vi "Shutdown.vi"(8 "error in (no error)":errorcluster, 11 "GRMActor in":refnum<class "GRMActor.lvclass">) -> (0 "error out":errorcluster, 3 "GRMActor out":refnum<class "GRMActor.lvclass">)   [LabVIEW 2020, in "GRMActor.lvlib" / "GRMActor.lvclass"]
uses:
  GRMActor.lvclass
  GRMActor.lvclass/GRMActor.ctl
  <vilib>/ActorFramework/Message Enqueuer/Message Enqueuer.lvclass/Message Enqueuer.ctl
  <vilib>/ActorFramework/Message Enqueuer/Enqueue.vi
  <vilib>/ActorFramework/Stop Msg/Stop Msg.lvclass
  C:/Program Files/National Instruments/LabVIEW 2020/vi.lib/ActorFramework/Message/Message.lvclass
  <vilib>/ActorFramework/Message Priority Queue/Priority Enqueue.vi
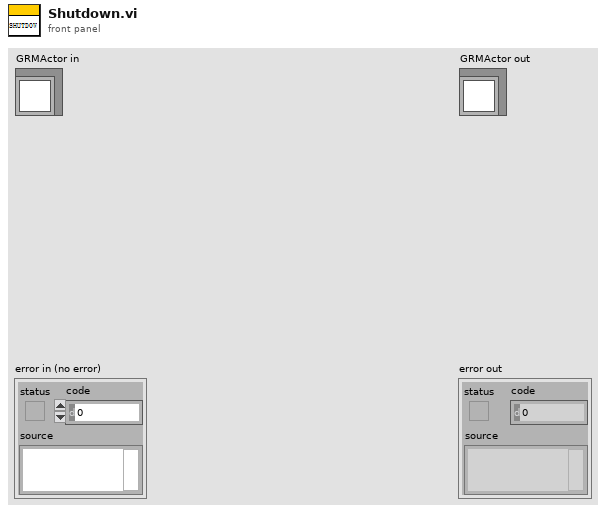
[diagram p1: front panel]
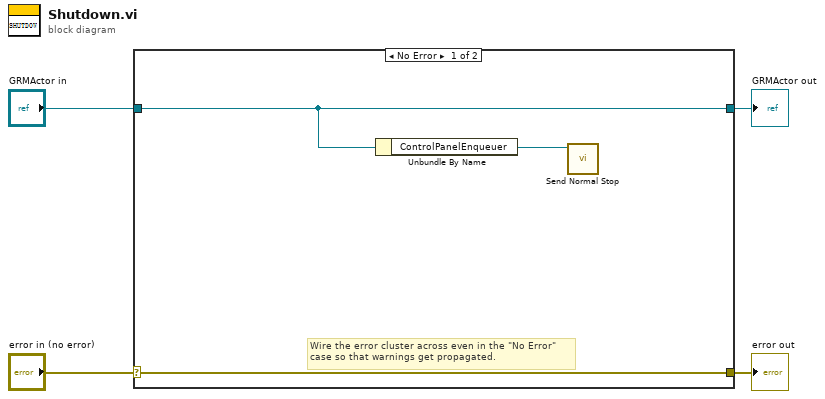
[diagram p0: block diagram]
diagram:
  n1 = case shown="No Error" "error in (no error)" {
    selector: "error in (no error)" -> [w7 w9]
    tunnel: [w7 w9] -> w3
    tunnel: [w6 w8] -> w1
    tunnel: "GRMActor in" -> [w6 w8]
    frame No Error {
      # "Wire the error cluster across even in the \"No Error\"\ncase so that warnings get propagated."
      n2 = Unbundle By Name(w6) -> ("ControlPanelEnqueuer"=w5:refnum<class "Message Enqueuer.lvclass">)
      n3 = call <vilib>:"Send Normal Stop.vi"("Message Enqueuer"=w5) -> ()  [unwired: 10 in, 1 out]
    }
    frame Error {
    }
  }
  "error out" <- w3
  "GRMActor out" <- w1
